vi "CAN Jaguar Get Version.vi"(8 "error in (no error)":errorcluster, 11 "CAN Jaguar Ref":T1={"Device Number"=0, "Control Mode"=enum."Percent VBus", "Inverted"=FALSE, "Semaphore"=refnum, "Max Vout"=12.0, "DevStatus"={"status"=FALSE, "code"=0, "source"=""}}) -> (0 "error out":errorcluster, 1 "Hardware Version":u8, 2 "Firmware Version":u32, 3 "CAN Jaguar Ref Out":T1={"Device Number"=0, "Control Mode"=enum."Percent VBus", "Inverted"=FALSE, "Semaphore"=refnum, "Max Vout"=12.0, "DevStatus"={"status"=FALSE, "code"=0, "source"=""}})   [LabVIEW 2009, in "CAN.lvlib"]
uses:
  CAN.lvlib
  CAN System Message IDs.ctl
  CAN Update Message IDs.ctl
  CAN Jaguar Control Mode.ctl
  CAN Jaguar Ref.ctl
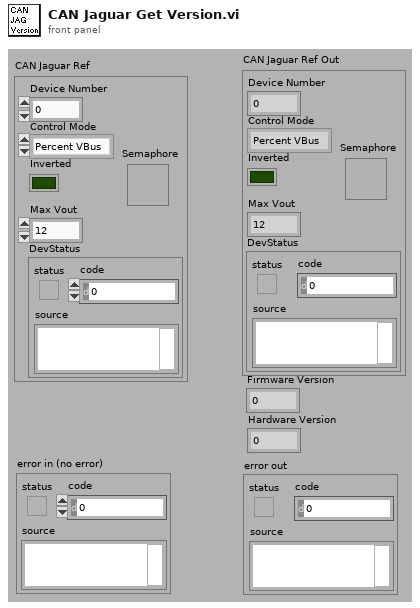
[diagram p1: front panel]
types:
  T1 = typedef "CAN.lvlib/CAN Jaguar Ref.ctl" = cluster{"Device Number":u8, "Control Mode":T2, "Inverted":bool, "Semaphore":T3, "Max Vout":dbl, "DevStatus":errorcluster}
  T2 = typedef "CAN.lvlib/CAN Jaguar Control Mode.ctl" = enum16{"Percent VBus", "Speed", "Position", "Current"}
  T3 = typedef "Semaphore RefNum" = refnum<k1>
  T4 = enum16{"big-endian, network order", "native, host order", "little-endian"}
  T5 = typedef "CAN.lvlib/CAN System Message IDs.ctl" = u32
  T6 = typedef "CAN.lvlib/CAN Update Message IDs.ctl" = u32
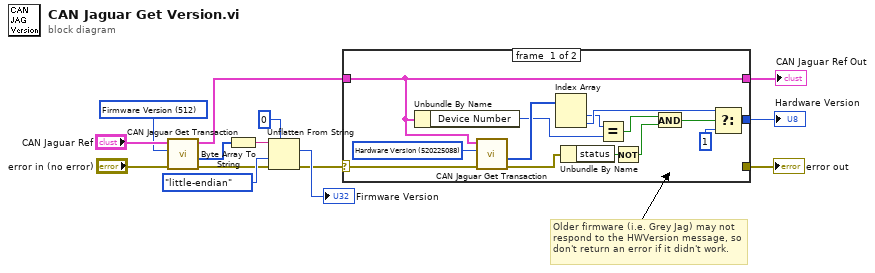
[diagram p0: block diagram]
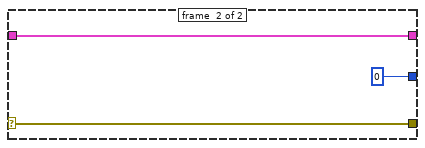
[diagram p2: hidden frame]
diagram:
  w6 = T5 512 items=["Device Assignment"=128, "Device Query"=192, "Sync Update"=384, "Firmware Update"=448, "Firmware Version"=512, "Enumerate"=576] ("CAN System Message IDs")
  # "Older firmware (i.e. Grey Jag) may not respond to the HWVersion message, so don't return an error if it didn't work."
  n1 = call "CAN Jaguar Get Transaction.vi"("error in"="error in (no error)", "Message ID"=w6, "CAN Jaguar Ref"="CAN Jaguar Ref") -> ("error out"=w4:errorcluster, "Data"=w1:u8[], "CAN Jaguar Ref Out"=w3:T1)  [unwired: 6 out]
  n2 = Byte Array To String(unsigned byte array=w1) -> (string=w14:string)
  n3 = Unflatten From String(type=u32 0, binary string=w14, byte order (0:big-endian, network order)=T4."little-endian", error in (no error)=w4) -> (value=→"Firmware Version":u32, error out=w8:errorcluster)  [unwired: 2 out]
  n4 = case shown="Error" w8 {
    selector: w8 -> [w19 w31]
    tunnel: [_ w31] -> w10
    tunnel: [w24 u8 0 ("f")] -> w9
    tunnel: w3 -> [w16 w29]
    tunnel: [w16 w29] -> w2
    frame #0 {
      w20 = T6 520225088 items=["Update Ping"=520224768, "Update Download"=520224832, "Update Send Data"=520224896, "Update Reset"=520224960, "Update Acknowledge"=520225024, "Hardware Version"=520225088] ("CAN Update Message IDs")
      n5 = Unbundle By Name(w16) -> ("Device Number"=w15:u8)
      n6 = call "CAN Jaguar Get Transaction.vi"("error in"=w19, "Message ID"=w20, "CAN Jaguar Ref"=w16) -> ("error out"=w18:errorcluster, "Data"=w17:u8[])  [unwired: 7 out]
      n7 = Index Array(array=w17) -> (element #1=w27:u8, element #2=w28:u8)  [unwired: 2 in]
      n8 = Unbundle By Name(w18) -> ("status"=w23:bool)
      n9 = Equal?(x=w27, y=w15) -> (x = y?=w26:bool)
      n10 = Not(x=w23) -> (.not. x?=w21:bool)
      n11 = And(x=w26, y=w21) -> (x .and. y?=w22:bool)
      n12 = Select(t=w28, s=w22, f=u8 1) -> (s? t:f=w24:u8)
    }
    frame #1 {
    }
  }
  "error out" <- w10
  "Hardware Version" <- w9
  "CAN Jaguar Ref Out" <- w2
